vi "Read Samples (Interleaved IQ Bytes).vi"(8 "error in (no error)":errorcluster, 10 "Samples":i32, 11 "RTL-SDR in":refnum<class "Session.lvclass">) -> (0 "error out":errorcluster, 2 "Interleaved IQ Bytes":u8[](array[numeric]), 3 "RTL-SDR out":refnum<class "Session.lvclass">)   [LabVIEW 2021, in "RTL-SDR.lvlib" / "Session.lvclass"]
uses:
  Session.lvclass
  Session.lvclass/Session.ctl
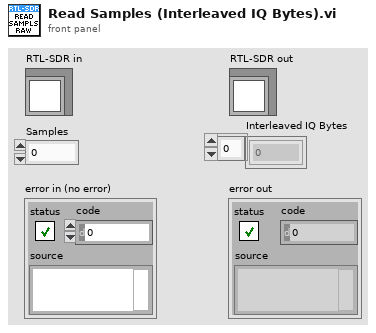
[diagram p1: front panel]
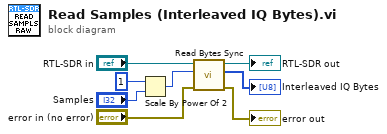
[diagram p0: block diagram]
diagram:
  n1 = Scale By Power Of 2(n=1, x="Samples") -> (x*2^n=w4:i32)
  n2 = call "Read Bytes Sync.vi"("error in (no error)"="error in (no error)", "len"=w4, "RTL-SDR in"="RTL-SDR in") -> ("error out"=→"error out":errorcluster, "buf"=→"Interleaved IQ Bytes":u8[], "RTL-SDR out"=→"RTL-SDR out":refnum<class "Session.lvclass">)  [unwired: 6 in]
